vi "Alignment.vi"(0 "Range":dbl=25.0 format="%#_13g", 1 "Camera Feedback":dbl=-244.57472985881094 format="%#_13g", 2 "Target":dbl format="%#_13g", 3 "POV":i32=180, 4 "Max Error":dbl=100.0 format="%#_13g", 5 "Effort Addition":dbl=0.175 min=0.0 max=1.0 step=0.05 format="%#_13g", 9 "Turn_Gain":dbl=0.25 format="%#_13g") -> (14 "Right Motor":dbl=0.425 format="%#_13g", 15 "Left Motor":dbl=-0.425 format="%#_13g", 17 "LeftAndRight?":bool)   [LabVIEW 2016]
panel:
  in  "LeftMotorSpeed":dbl format="%#_13g"
  in  "RightMotorSpeed":dbl format="%#_13g"
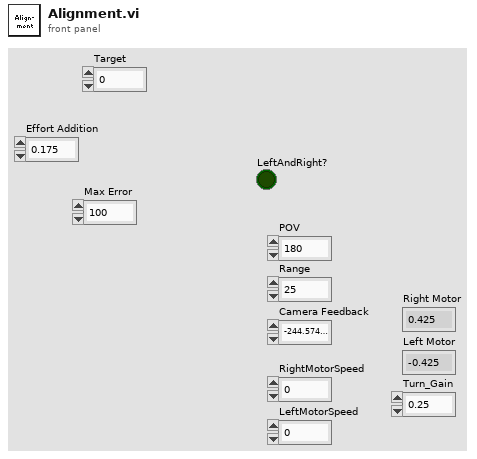
[diagram p1: front panel]
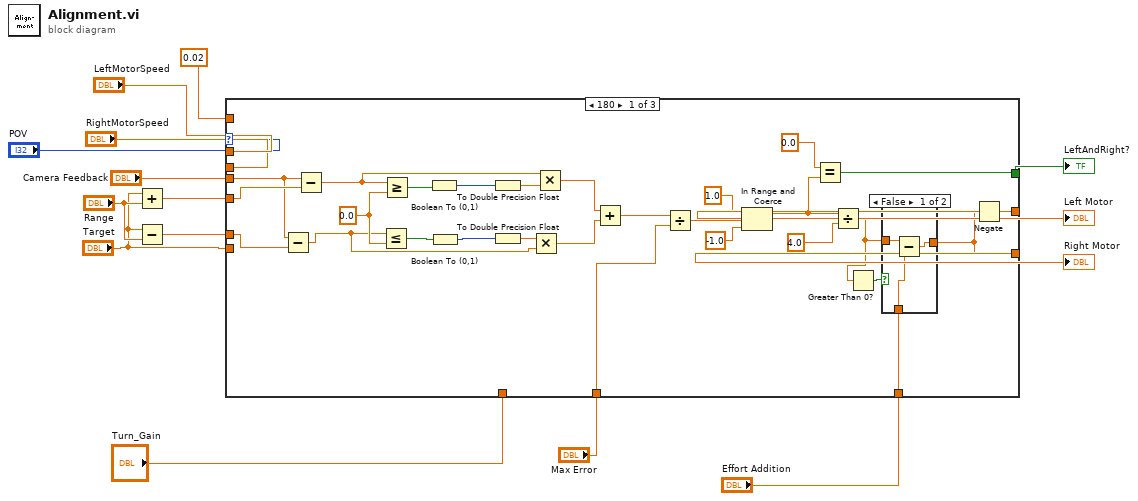
[diagram p0: block diagram]
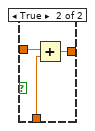
[diagram p2: hidden frame]
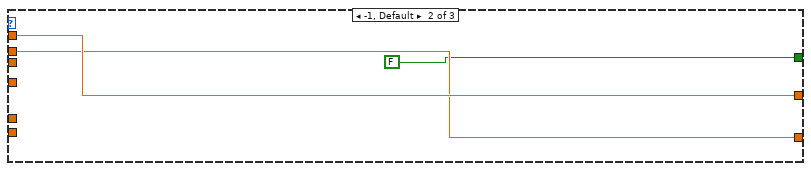
[diagram p3: hidden frame]
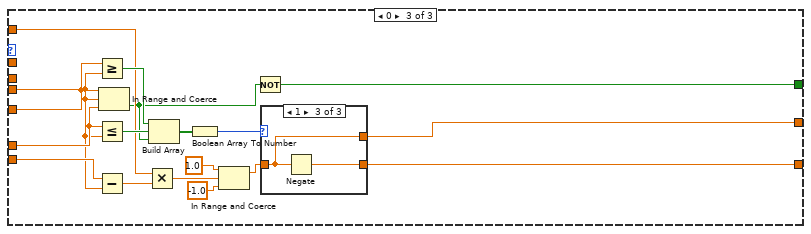
[diagram p4: hidden frame]
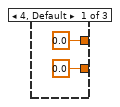
[diagram p5: hidden frame]
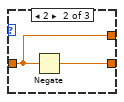
[diagram p6: hidden frame]
diagram:
  n1 = Add(x="Target", y="Range") -> (x+y=w9:dbl)
  n2 = Subtract(x="Target", y="Range") -> (x-y=w8:dbl)
  n3 = case shown="180" "POV" {
    tunnel: [w17 w52 w66] -> w15
    tunnel: "LeftMotorSpeed" -> [_ w52 _]
    tunnel: [w18 w51 w67] -> w13
    tunnel: "RightMotorSpeed" -> [_ w51 _]
    tunnel: "Camera Feedback" -> [w42 _ w61]
    tunnel: w9 -> [w43 _ w65]
    tunnel: w8 -> [w41 _ w70]
    tunnel: [w29 FALSE w53] -> w6
    tunnel: "Target" -> [_ _ w62]
    tunnel: 0.02 -> [_ _ w59]
    tunnel: "Turn_Gain" -> [_ _ _]
    tunnel: "Effort Addition" -> [w19 _ _]
    tunnel: "Max Error" -> [w16 _ _]
    frame 180 {
      w40 = 0.0
      n4 = Subtract(x=w42, y=w41) -> (x-y=w36:dbl)
      n5 = Subtract(x=w42, y=w43) -> (x-y=w38:dbl)
      n6 = Less Or Equal?(x=w36, y=w40) -> (x <= y?=w23:bool)
      n7 = Greater Or Equal?(x=w38, y=w40) -> (x >= y?=w21:bool)
      n8 = Boolean To (0,1)(Boolean=w21) -> (0, 1=w20:i16)
      n9 = Boolean To (0,1)(Boolean=w23) -> (0, 1=w22:i16)
      n10 = To Double Precision Float(number=w20) -> (double precision float=w39:dbl)
      n11 = To Double Precision Float(number=w22) -> (double precision float=w37:dbl)
      n12 = Multiply(x=w37, y=w36) -> (x*y=w34:dbl)
      n13 = Multiply(x=w38, y=w39) -> (x*y=w35:dbl)
      n14 = Add(x=w35, y=w34) -> (x+y=w33:dbl)
      n15 = Divide(x=w33, y=w16) -> (x/y=w32:dbl)
      n16 = In Range and Coerce(upper limit=1.0, x=w32, lower limit=-1.0) -> (coerced(x)=w27:dbl)  [unwired: 1 out]
      n17 = Equal?(x=0.0, y=w27) -> (x = y?=w29:bool)
      n18 = Divide(x=w27, y=4.0) -> (x/y=w24:dbl)
      n19 = Greater Than 0?(x=w24) -> (x > 0?=w25:bool)
      n20 = case shown="False" w25 {
        tunnel: w24 -> [w46 w49]
        tunnel: [w45 w48] -> w18
        tunnel: w19 -> [w44 w47]
        frame False {
          n21 = Subtract(x=w46, y=w44) -> (x-y=w45:dbl)
        }
        frame True {
          n22 = Add(x=w49, y=w47) -> (x+y=w48:dbl)
        }
      }
      n23 = Negate(x=w18) -> (-x=w17:dbl)
    }
    frame -1, Default {
    }
    frame 0 {
      n24 = Greater Or Equal?(x=w65, y=w61) -> (x >= y?=w64:bool)
      n25 = Less Or Equal?(x=w70, y=w61) -> (x <= y?=w63:bool)
      n26 = Subtract(x=w62, y=w61) -> (x-y=w60:dbl)
      n27 = In Range and Coerce(upper limit=w65, x=w61, lower limit=w70) -> (In Range?=w54:bool)  [unwired: 1 out]
      n28 = Multiply(x=w59, y=w60) -> (x*y=w58:dbl)
      n29 = Build Array(w64, w63, w54) -> (w69:bool[])
      n30 = Boolean Array To Number(Boolean array=w69) -> (number=w68:u32)
      n31 = In Range and Coerce(upper limit=1.0, x=w58, lower limit=-1.0) -> (coerced(x)=w57:dbl)  [unwired: 1 out]
      n32 = Not(x=w54) -> (.not. x?=w53:bool)
      n33 = case shown="1" w68 {
        tunnel: [0.0 w73 w75] -> w67
        tunnel: [0.0 w74 w76] -> w66
        tunnel: w57 -> [_ w74 w76]
        frame 4, Default {
        }
        frame 2 {
          n34 = Negate(x=w74) -> (-x=w73:dbl)
        }
        frame 1 {
          n35 = Negate(x=w76) -> (-x=w75:dbl)
        }
      }
    }
  }
  "Left Motor" <- w15
  "Right Motor" <- w13
  "LeftAndRight?" <- w6
